vi "Get File Statistics.vi"(8 "error in (no error)":errorcluster, 10 "Simple Read":bool, 11 "Read Write BLF in":refnum<class "Read Write BLF.lvclass">) -> (0 "error out":errorcluster, 1 "Objecs Read Position":u32, 2 "Object Count":u32, 3 "Read Write BLF out":refnum<class "Read Write BLF.lvclass">, 4 "Last Object Time":timestamp, 5 "Application Information":T1, 6 "Start Time":timestamp)   [LabVIEW 2015, in "Read Write BLF.lvclass"]
doc: "This VI will return the file statistics for a BLF file. This includes things like the number of Objects in the file, the current read position, information about the application that made the file, and the time that the first, and last objects were written.\n\n-------------\nBrian Hoover (Hooovahh)"
uses:
  Read Write BLF.lvclass
  Controls/Cluster - Application Information.ctl
  Controls/Enum - Application ID.ctl
  Read Write BLF.lvclass/Read Write BLF.ctl
  Controls/Cluster - VBLFileStatisticsEx.ctl
  Controls/Cluster - SystemTime.ctl
  <vilib>/Utility/miscctls.llb/LVDateTimeRec.ctl
  Controls/Cluster - VBLFileStatistics.ctl
  <vilib>/Utility/error.llb/Error Cluster From Error Code.vi
  <vilib>/Utility/file.llb/Application Directory.vi
  <vilib>/ErrorRing/Error Ring.xnode
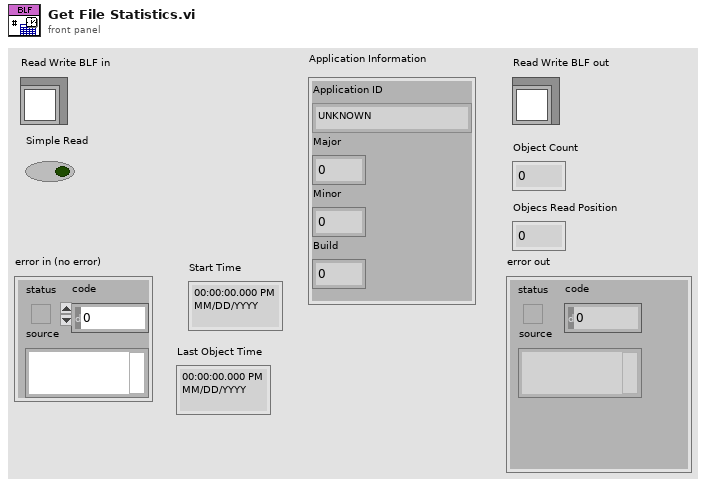
[diagram p1: front panel]
types:
  T1 = typedef "Read Write BLF.lvclass/Cluster - Application Information.ctl" = cluster{"Application ID":T2, "Major":u8, "Minor":u8, "Build":u8}
  T2 = typedef "Read Write BLF.lvclass/Enum - Application ID.ctl" = enum8{"UNKNOWN", "CANALYZER", "CANOE", "CANSTRESS", "CANLOG", "CANAPE", "CANCASEXLLOG"}
  T3 = typedef "LVDateTimeRec.ctl" = cluster{"fractional second":dbl, "second":i32, "minute":i32, "hour":i32, "day of month":i32, "month":i32, "year":i32, "day of week":i32, "day of year":i32, "DST":i32}
  T4 = typedef "Read Write BLF.lvclass/Cluster - VBLFileStatisticsEx.ctl" = cluster{"mStatisticSize":u32, "Application ID":T2, "mApplicationMajor":u8, "mApplicationMinor":u8, "mApplicationBuild":u8, "mFileSize":u64, "mUncompressedFileSize":u64, "mObjectCount":u32, "mObjectsRead":u32, "mMeasurementStartTime ":T5, "mLastObjectTime":T5, "mReserved":cluster{"mReserved[0]":u32, "mReserved[1]":u32, "mReserved[2]":u32, "mReserved[3]":u32, "mReserved[4]":u32, "mReserved[5]":u32, "mReserved[6]":u32, "mReserved[7]":u32, "mReserved[8]":u32, "mReserved[9]":u32, "mReserved[10]":u32, "mReserved[11]":u32, "mReserved[12]":u32, "mReserved[13]":u32, "mReserved[14]":u32, "mReserved[15]":u32, "mReserved[16]":u32, "mReserved[17]":u32}}
  T5 = typedef "Read Write BLF.lvclass/Cluster - SystemTime.ctl" = cluster{"Year":u16, "Month":u16, "DayOfWeek":u16, "Day":u16, "Hour":u16, "Minute":u16, "Second":u16, "Milliseconds":u16}
  T6 = typedef "Read Write BLF.lvclass/Cluster - VBLFileStatistics.ctl" = cluster{"mStatisticSize":u32, "Application ID":T2, "mApplicationMajor":u8, "mApplicationMinor":u8, "mApplicationBuild":u8, "mFileSize":u64, "mUncompressedFileSize":u64, "mObjectCount":u32, "mObjecsRead":u32}
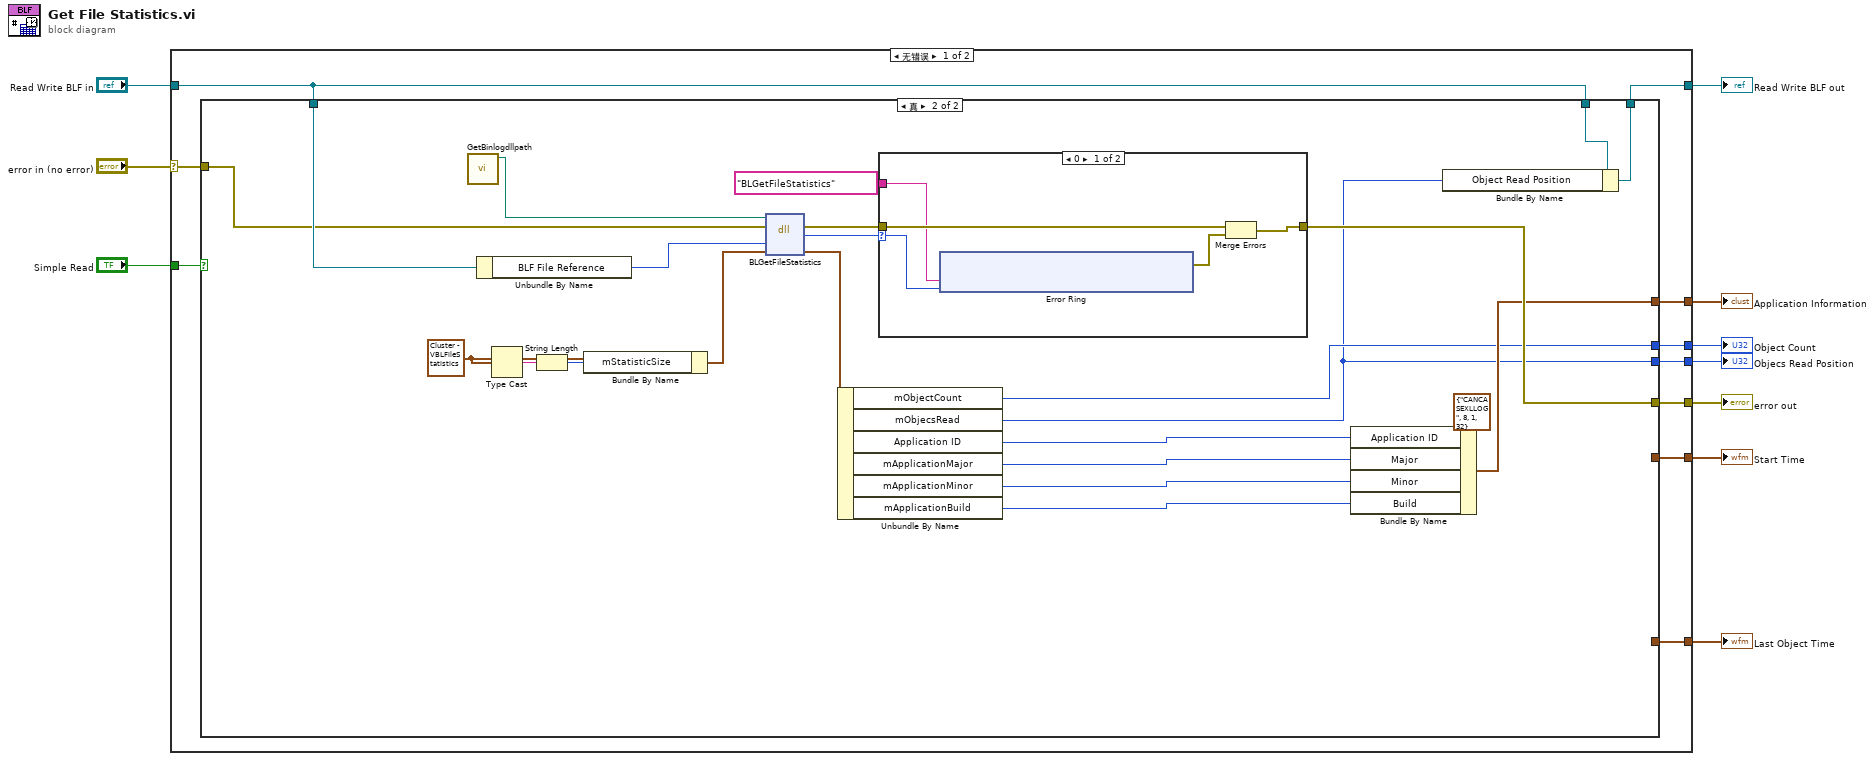
[diagram p0: block diagram]
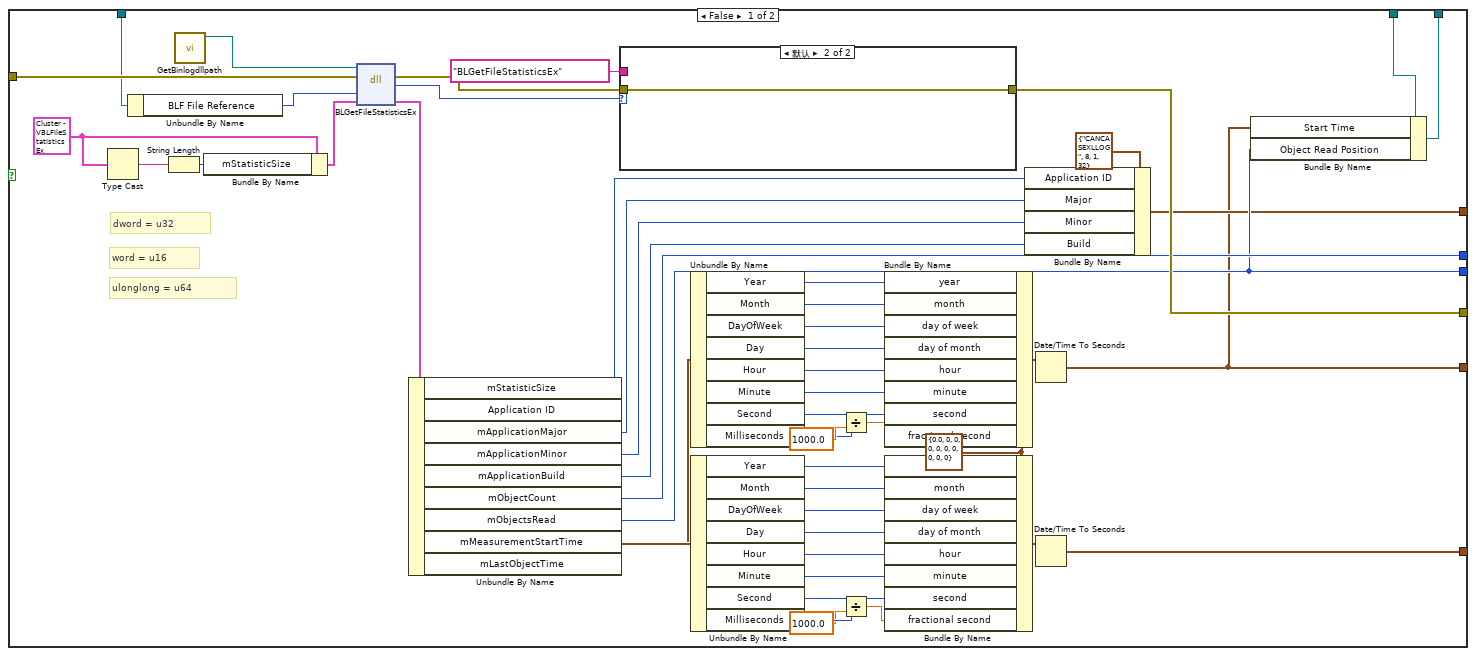
[diagram p2: hidden frame]
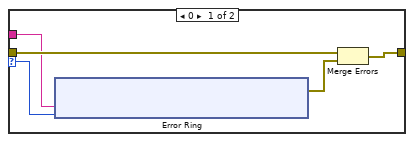
[diagram p3: hidden frame]
diagram:
  n1 = case shown="无错误" "error in (no error)" {
    selector: "error in (no error)" -> [w20 w123]
    tunnel: [w19 w123] -> w9
    tunnel: [w16 w122] -> w7
    tunnel: "Read Write BLF in" -> [w12 w122]
    tunnel: [w13 _] -> w6
    tunnel: [w18 _] -> w5
    tunnel: [w17 _] -> w4
    tunnel: [w15 _] -> w3
    tunnel: [w14 _] -> w2
    tunnel: "Simple Read" -> [w11 _]
    frame No Error {
      n2 = case shown="真" w11 {
        tunnel: w12 -> [w70 w97]
        tunnel: w20 -> [w69 w98]
        tunnel: [w68 w94] -> w19
        tunnel: [w67 _] -> w18
        tunnel: [w66 w87] -> w17
        tunnel: [w65 w96] -> w16
        tunnel: [w64 w86] -> w15
        tunnel: [w63 w88] -> w14
        tunnel: [w62 _] -> w13
        tunnel: w12 -> [w22 w99]
        frame False {
          w29 = T3 {"fractional second"=0.0, "second"=0, "minute"=0, "hour"=0, "day of month"=0, "month"=0, "year"=0, "day of week"=0, "day of year"=0, "DST"=0} ("date time rec")
          w54 = T4 {"mStatisticSize"=0, "Application ID"=enum."UNKNOWN", "mApplicationMajor"=0, "mApplicationMinor"=0, "mApplicationBuild"=0, "mFileSize"=0, "mUncompressedFileSize"=0, "mObjectCount"=0, "mObjectsRead"=0, "mMeasurementStartTime "={"Year"=1988, "Month"=4, "DayOfWeek"=5, "Day"=13, "Hour"=12, "Minute"=12, "Second"=12, "Milliseconds"=0}, "mLastObjectTime"={"Year"=1988, "Month"=4, "DayOfWeek"=5, "Day"=13, "Hour"=12, "Minute"=12, "Second"=12, "Milliseconds"=0}, "mReserved"={"mReserved[0]"=0, "mReserved[1]"=0, "mReserved[2]"=0, "mReserved[3]"=0, "mReserved[4]"=0, "mReserved[5]"=0, "mReserved[6]"=0, "mReserved[7]"=0, "mReserved[8]"=0, "mReserved[9]"=0, "mReserved[10]"=0, "mReserved[11]"=0, "mReserved[12]"=0, "mReserved[13]"=0, "mReserved[14]"=0, "mReserved[15]"=0, "mReserved[16]"=0, "mReserved[17]"=0}}
          # "ulonglong = u64"
          # "word = u16"
          # "dword = u32"
          n3 = Type Cast(x=w54) -> (*(type *) &x=w57:string)  [unwired: 1 in]
          n4 = Unbundle By Name(w22) -> ("BLF File Reference"=w61:u32)
          n5 = String Length(string=w57) -> (length=w55:i32)
          n6 = call "GetBinlogdllpath.vi"() -> ("dup path"=w21:path)  [unwired: 11 in]
          n7 = Bundle By Name(cluster=w54, "mStatisticSize"=w55) -> (w56:T4)
          n8 = dll-call lib="PTH2Xabs E自开发软件X-CAN项目 X-CAN离线分析平台 V2.2.8.0BLF\nbinlog.dll" fn="BLGetFileStatisticsEx"(path in=w21, error in=w69, "hFile"=w61, "pStatistics"=w56) -> (error out=w58:errorcluster, "return type"=w59:i32, "pStatistics"=w53:T4)  [unwired: 2 in, 1 out]
          n9 = Unbundle By Name(w53) -> ("Application ID"=w26:T2, "mApplicationMajor"=w25:u8, "mApplicationMinor"=w24:u8, "mApplicationBuild"=w23:u8, "mObjectCount"=w66:u32, "mObjectsRead"=w64:u32, "mMeasurementStartTime"=w28:T5, "mLastObjectTime"=w52:T5)  [unwired: 1 out]
          n10 = case shown="默认" w59 {
            selector: w59 -> [w73 _]
            tunnel: w58 -> [w75 w84]
            tunnel: [w74 w84] -> w68
            tunnel: "BLGetFileStatisticsEx" -> [w72 _]
            frame 0 {
              n11 = xnode "Error Ring"("参数 0"=w72, "参数 1"=w73) -> ("错误输出"=w71:errorcluster)
              n12 = Merge Errors(w75, w71) -> (w74:errorcluster)
            }
            frame Default {
            }
          }
          n13 = Unbundle By Name(w28) -> ("Year"=w31:u16, "Month"=w32:u16, "DayOfWeek"=w33:u16, "Day"=w34:u16, "Hour"=w35:u16, "Minute"=w36:u16, "Second"=w37:u16, "Milliseconds"=w38:u16)
          n14 = Unbundle By Name(w52) -> ("Year"=w50:u16, "Month"=w49:u16, "DayOfWeek"=w48:u16, "Day"=w47:u16, "Hour"=w46:u16, "Minute"=w45:u16, "Second"=w44:u16, "Milliseconds"=w43:u16)
          n15 = Divide(x=w38, y=1000.0) -> (x/y=w40:dbl)
          n16 = Divide(x=w43, y=1000.0) -> (x/y=w41:dbl)
          n17 = Bundle By Name(cluster=w29, "year"=w31, "month"=w32, "day of week"=w33, "day of month"=w34, "hour"=w35, "minute"=w36, "second"=w37, "fractional second"=w40) -> (w30:T3)
          n18 = Bundle By Name(cluster=w29, "year"=w50, "month"=w49, "day of week"=w48, "day of month"=w47, "hour"=w46, "minute"=w45, "second"=w44, "fractional second"=w41) -> (w51:T3)
          n19 = Bundle By Name(cluster=T1 {"Application ID"=enum."CANCASEXLLOG", "Major"=8, "Minor"=1, "Build"=32}, "Application ID"=w26, "Major"=w25, "Minor"=w24, "Build"=w23) -> (w63:T1)
          n20 = Date/Time To Seconds(2:w30) -> (0:w62:timestamp)  [unwired: 1 in]
          n21 = Date/Time To Seconds(2:w51) -> (0:w67:timestamp)  [unwired: 1 in]
          n22 = Bundle By Name(cluster=w70, "Start Time"=w62, "Object Read Position"=w64) -> (w65:refnum<class "Read Write BLF.lvclass">)
        }
        frame True {
          w102 = T6 {"mStatisticSize"=0, "Application ID"=enum."UNKNOWN", "mApplicationMajor"=0, "mApplicationMinor"=0, "mApplicationBuild"=0, "mFileSize"=0, "mUncompressedFileSize"=0, "mObjectCount"=0, "mObjecsRead"=0}
          n23 = call "GetBinlogdllpath.vi"() -> ("dup path"=w85:path)  [unwired: 11 in]
          n24 = Unbundle By Name(w99) -> ("BLF File Reference"=w107:u32)
          n25 = Type Cast(x=w102) -> (*(type *) &x=w101:string)  [unwired: 1 in]
          n26 = String Length(string=w101) -> (length=w100:i32)
          n27 = Bundle By Name(cluster=w102, "mStatisticSize"=w100) -> (w103:T6)
          n28 = dll-call lib="PTH2Xabs E自开发软件X-CAN项目 X-CAN离线分析平台 V2.2.8.0BLF\nbinlog.dll" fn="BLGetFileStatistics"(path in=w85, error in=w98, "hFile"=w107, "pStatistics"=w103) -> (error out=w104:errorcluster, "return type"=w105:i32, "pStatistics"=w95:T6)  [unwired: 2 in, 1 out]
          n29 = Unbundle By Name(w95) -> ("mObjectCount"=w87:u32, "mObjecsRead"=w86:u32, "Application ID"=w92:T2, "mApplicationMajor"=w91:u8, "mApplicationMinor"=w90:u8, "mApplicationBuild"=w89:u8)
          n30 = case shown="0" w105 {
            selector: w105 -> [w110 _]
            tunnel: w104 -> [w112 w121]
            tunnel: [w111 w121] -> w94
            tunnel: "BLGetFileStatistics" -> [w109 _]
            frame 0 {
              n31 = xnode "Error Ring"("参数 0"=w109, "参数 1"=w110) -> ("错误输出"=w108:errorcluster)
              n32 = Merge Errors(w112, w108) -> (w111:errorcluster)
            }
            frame Default {
            }
          }
          n33 = Bundle By Name(cluster=T1 {"Application ID"=enum."CANCASEXLLOG", "Major"=8, "Minor"=1, "Build"=32}, "Application ID"=w92, "Major"=w91, "Minor"=w90, "Build"=w89) -> (w88:T1)
          n34 = Bundle By Name(cluster=w97, "Object Read Position"=w86) -> (w96:refnum<class "Read Write BLF.lvclass">)
        }
      }
    }
    frame Error {
    }
  }
  "error out" <- w9
  "Read Write BLF out" <- w7
  "Start Time" <- w6
  "Last Object Time" <- w5
  "Object Count" <- w4
  "Objecs Read Position" <- w3
  "Application Information" <- w2
